vi "NameFileAndFolder.vi"(2 "ext":string="*.pos", 3 "Head Directory":string="d:\\calibration\\position_defl") -> (0 "New Filename":string, 1 "Sub Directory":string="d:\\calibration\\position_defl")   [LabVIEW 2012]
panel:
  out "New Directory":bool
  out "File num":i32
  out "Current Files":string[](array[string])
  # "Name File And Folder"
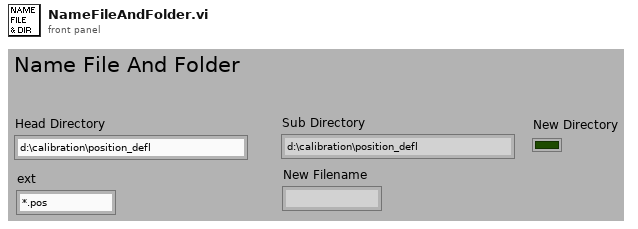
[diagram p1: front panel]
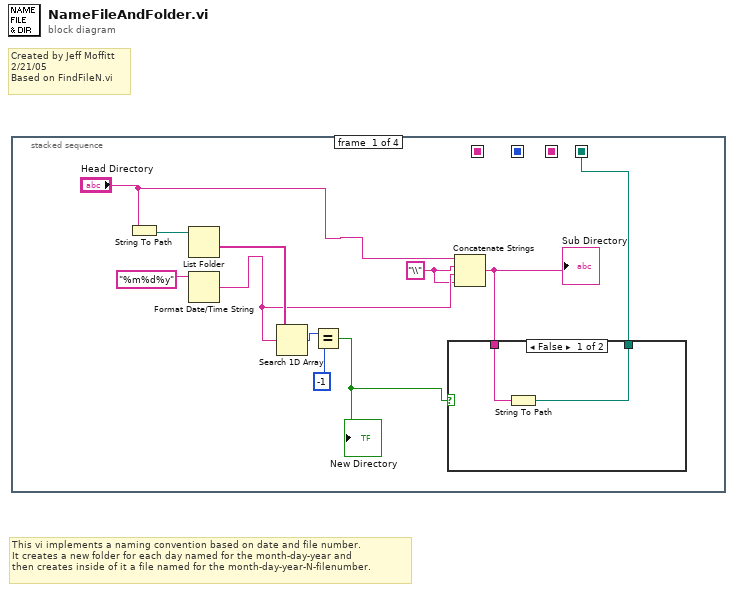
[diagram p0: block diagram]
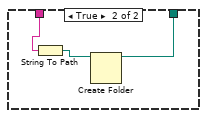
[diagram p2: hidden frame]
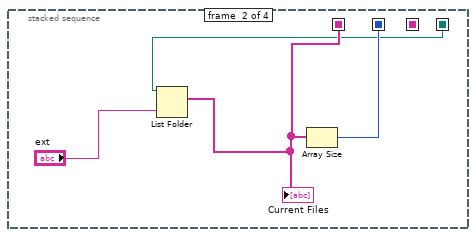
[diagram p3: hidden frame]
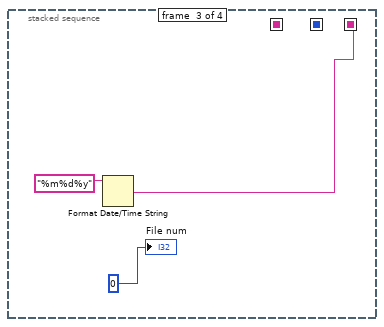
[diagram p4: hidden frame]
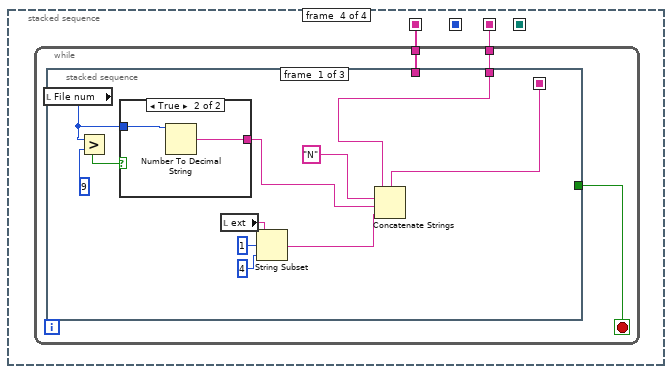
[diagram p5: hidden frame]
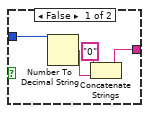
[diagram p6: hidden frame]
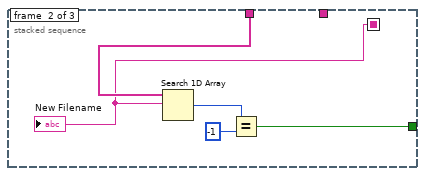
[diagram p7: hidden frame]
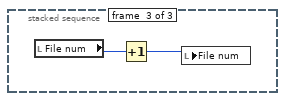
[diagram p8: hidden frame]
diagram:
  # "This vi implements a naming convention based on date and file number.\nIt creates a new folder for each day named for the month-day-year and\nthen creates inside of it a file named for the month-day-year-N-filenumber."
  # "Created by Jeff Moffitt\n2/21/05\nBased on FindFileN.vi"
  n1 = stacked-sequence {
    seq-local: [_ w19 _ _] -> [_ _ _ _]
    seq-local: [_ w18 _ _] -> [_ _ _ w24]
    seq-local: [_ _ w21 _] -> [_ _ _ w25]
    seq-local: [w1 _ _ _] -> [_ w17 _ _]
    frame #0 {
      w4 = "\\"
      n2 = String To Path(string="Head Directory") -> (path=w11:path)
      n3 = List Folder(path=w11) -> (folder names=w9:string[])  [unwired: 3 in, 3 out]
      n4 = Format Date/Time String(time format string (%c)="%m%d%y") -> (date/time string=w6:string)  [unwired: 2 in]
      n5 = Search 1D Array(1D array=w9, element=w6) -> (index of element=w8:i32)  [unwired: 1 in]
      n6 = Equal?(x=w8, y=-1) -> (x = y?=w3:bool)
      "New Directory" <- w3
      n7 = Concatenate Strings("Head Directory", w4, w6, w4) -> (w2:string)
      "Sub Directory" <- w2
      n8 = case shown="False" w3 {
        tunnel: w2 -> [w13 w16]
        tunnel: [w12 w14] -> w1
        frame False {
          n9 = String To Path(string=w13) -> (path=w12:path)
        }
        frame True {
          n10 = String To Path(string=w16) -> (path=w15:path)
          n11 = Create Folder(path (use dialog)=w15) -> (created path=w14:path)  [unwired: 2 in, 2 out]
        }
      }
    }
    frame #1 {
      n12 = List Folder(path=w17, pattern="ext") -> (filenames=w18:string[])  [unwired: 2 in, 3 out]
      "Current Files" <- w18
      n13 = Array Size(array=w18) -> (size(s)=w19:i32)
    }
    frame #2 {
      n14 = Format Date/Time String(time format string (%c)="%m%d%y") -> (date/time string=w21:string)  [unwired: 2 in]
      "File num" <- 0 ("File num")
    }
    frame #3 {
      n15 = while {
        tunnel: w24 -> [w27]
        tunnel: w25 -> [w28]
        stop <- w26 stop-if-true
        n16 = stacked-sequence {
          seq-local: [w33 _ _] -> [_ w49 _]
          tunnel: w28 -> [w39 _ _]
          tunnel: w27 -> [_ w50 _]
          tunnel: [_ w46 _] -> w26
          frame #0 {
            n17 = local read "File num"() -> (w35:i32)
            n18 = Greater?(x=w35, y=9) -> (0:w36:bool)
            n19 = case shown="True" w36 {
              tunnel: [w40 w45] -> w34
              tunnel: w35 -> [w43 w44]
              frame False {
                n20 = Number To Decimal String(number=w43) -> (decimal integer string=w41:string)  [unwired: 1 in]
                n21 = Concatenate Strings("0" ("Substring"), w41) -> (w40:string)
              }
              frame True {
                n22 = Number To Decimal String(number=w44) -> (decimal integer string=w45:string)  [unwired: 1 in]
              }
            }
            n23 = local read "ext"() -> (w32:string)
            n24 = String Subset(string=w32, offset (0)=1, length (rest)=4 ("length (rest)")) -> (substring=w29:string)
            n25 = Concatenate Strings(w39, "N" ("Substring"), w34, w29) -> (w33:string)
          }
          frame #1 {
            n26 = Search 1D Array(1D array=w50, element=w49) -> (index of element=w48:i32)  [unwired: 1 in]
            n27 = Equal?(x=w48, y=-1) -> (x = y?=w46:bool)
            "New Filename" <- w49
          }
          frame #2 {
            n28 = local read "File num"() -> (w52:i32)
            n29 = Increment(x=w52) -> (x+1=w51:i32)
            n30 = local write "File num"(w51) -> ()
          }
        }
      }
    }
  }
